vi "Point Dispense.vi"() -> ()   [LabVIEW 2016]
uses:
  GitHub/UCSB-Gantry/V5/Drivers/Aerotech A3200/Motion/WaitSingle.vi
  GitHub/UCSB-Gantry/V5/Drivers/Aerotech A3200/Aerotech VIs.lvlib
  GitHub/UCSB-Gantry/V5/Drivers/EFD Ultimus V/EFD Ultimus V.lvlib
panel:
  in  "stop":bool
  in  "Size of Square":dbl
  in  "Centerpoint":dbl[](array[numeric])
  in  "Go":bool
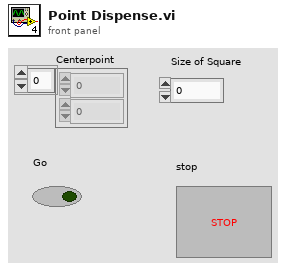
[diagram p1: front panel]
types:
  T1 = cluster{"Baud Rate ":u32, "Parity ":u16, "Data Bits ":u16, "Stop Bits":u16}
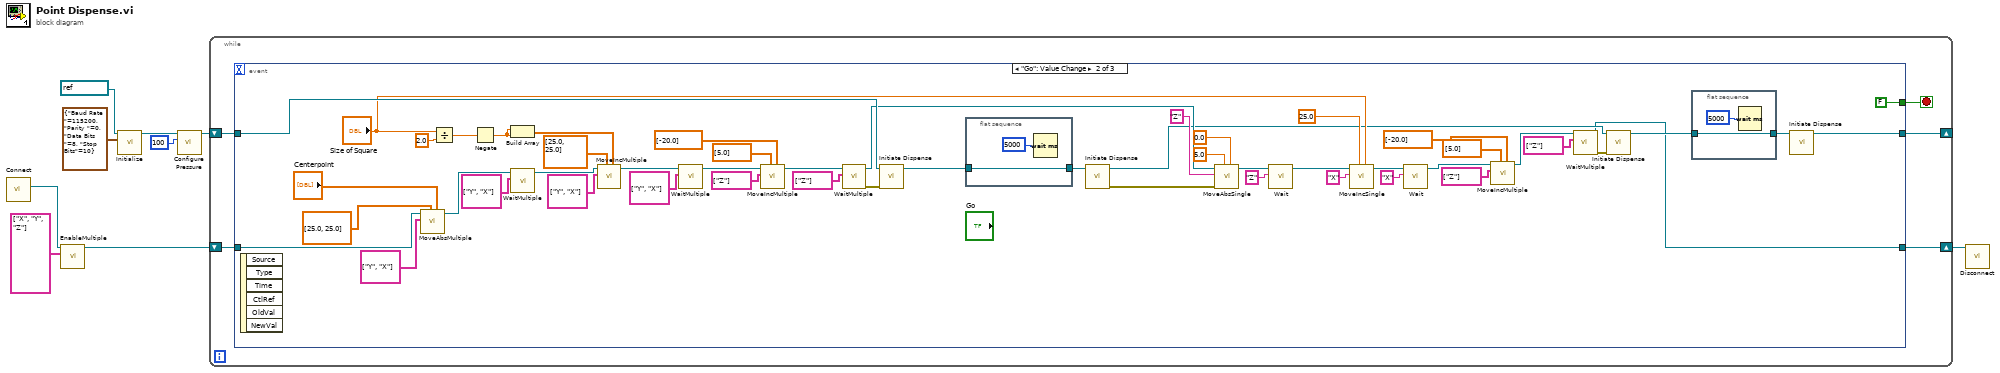
[diagram p0: block diagram]
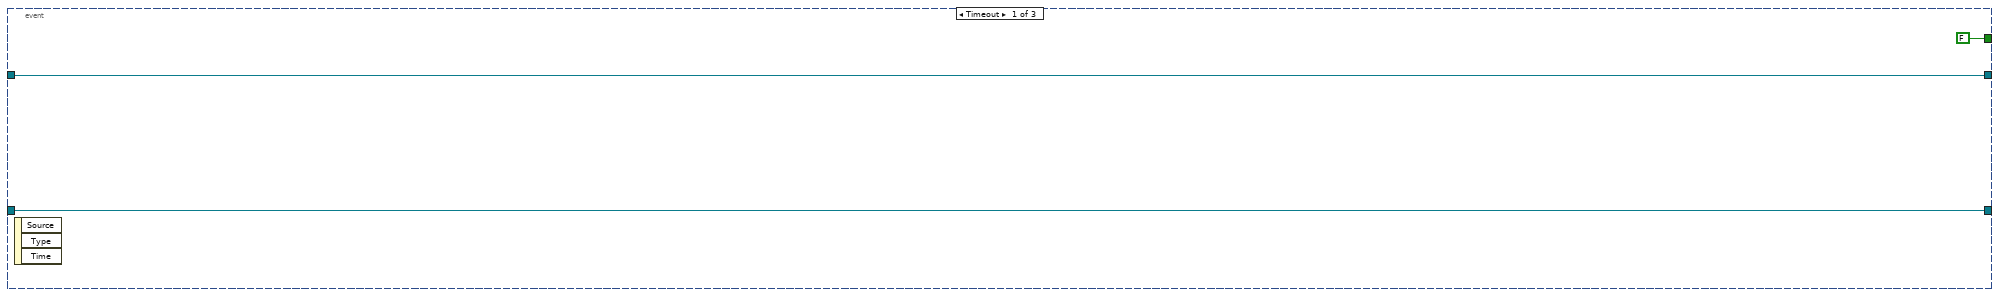
[diagram p2: hidden frame]
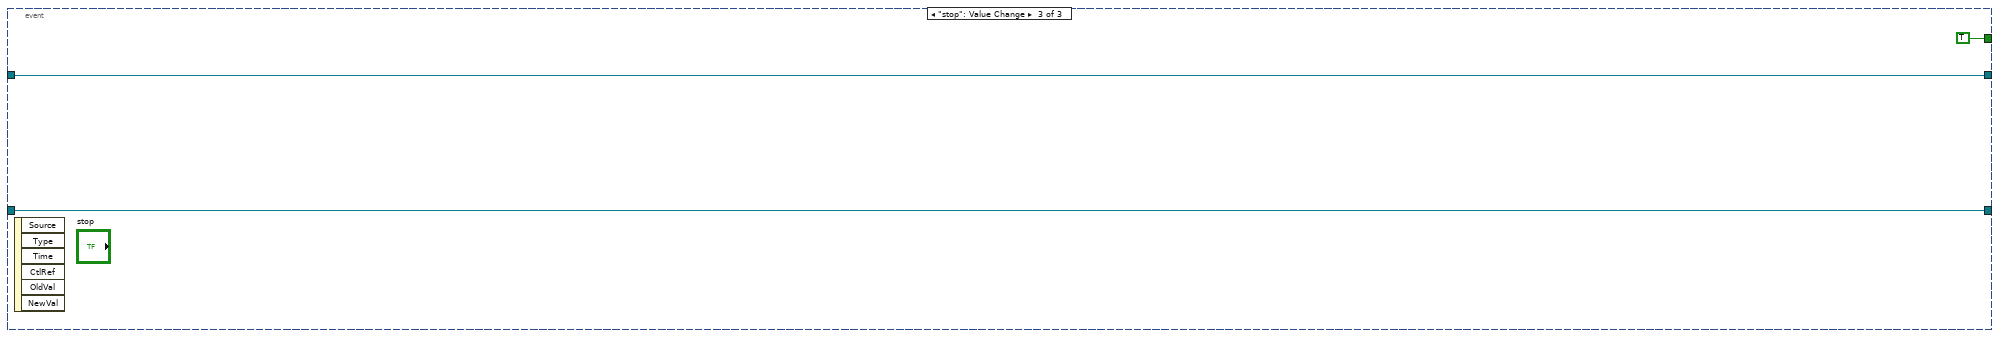
[diagram p3: hidden frame]
diagram:
  n1 = call "Connect.vi"() -> ("controller"=w9:refnum<k24>)  [unwired: 10 in, 1 out]
  n2 = call "EnableMultiple.vi"("axis names"=string[] ["X", "Y", "Z"], "controller in"=w9) -> ("controller out"=w7:refnum<k24>)  [unwired: 8 in, 1 out]
  n3 = call "Initialize.vi"("Serial Configuration"=T1 {"Baud Rate "=115200, "Parity "=0, "Data Bits "=8, "Stop Bits"=10}, "VISA resource name"=refnum<visa-resource-name> "COM1") -> ("VISA resource name out"=w3:refnum<visa-resource-name>)  [unwired: 8 in, 1 out]
  n4 = call "Configure Pressure.vi"("Pressure Setting (0000)"=i64 100, "VISA resource name"=w3) -> ("VISA resource name out"=w1:refnum<visa-resource-name>)  [unwired: 8 in, 1 out]
  n5 = while {
    shift-right: [w13] -> w6
    shift-left: w7 -> [w14]
    shift-right: [w10] -> _
    shift-left: w1 -> [w11]
    stop <- w12 stop-if-true
    n6 = event shown="[1] \"Go\": Value Change" {
      selector: _ -> [_ _ _]
      dyn-events: _ -> [_ _ _]
      timeout: _ -> [_ _ _]
      tunnel: w14 -> [w17 w66 w74]
      tunnel: [w17 w18 w74] -> w13
      tunnel: [FALSE FALSE TRUE] -> w12
      tunnel: w11 -> [w15 w46 w73]
      tunnel: [w15 w19 w73] -> w10
      event Timeout {
        n7 = event-data() -> ()  [unwired: 1 in, 3 out]
      }
      event "Go": Value Change {
        n8 = event-data() -> ()  [unwired: 1 in, 6 out]
        n9 = call "MoveAbsMultiple.vi"("positions"="Centerpoint", "speeds"=dbl[] [25.0, 25.0], "axis names"=string[] ["Y", "X"], "controller in"=w66) -> ("controller out"=w64:refnum<k24>)  [unwired: 6 in, 1 out]
        n10 = Divide(x="Size of Square", y=2.0) -> (x/y=w60:dbl)
        n11 = Negate(x=w60) -> (-x=w58:dbl)
        n12 = Build Array(w58, w58) -> (w57:dbl[])
        n13 = call "WaitMultiple.vi"("axis names"=string[] ["Y", "X"], "controller in"=w64) -> ("controller out"=w62:refnum<k24>)  [unwired: 7 in, 2 out]
        n14 = call "MoveIncMultiple.vi"("distances"=w57, "speeds"=dbl[] [25.0, 25.0], "axis names"=string[] ["Y", "X"], "controller in"=w62) -> ("controller out"=w54:refnum<k24>)  [unwired: 6 in, 1 out]
        n15 = call "WaitMultiple.vi"("axis names"=string[] ["Y", "X"], "controller in"=w54) -> ("controller out"=w52:refnum<k24>)  [unwired: 7 in, 2 out]
        n16 = call "MoveIncMultiple.vi"("distances"=dbl[] [-20.0], "speeds"=dbl[] [5.0], "axis names"=string[] ["Z"], "controller in"=w52) -> ("controller out"=w48:refnum<k24>)  [unwired: 6 in, 1 out]
        n17 = call "WaitMultiple.vi"("axis names"=string[] ["Z"], "controller in"=w48) -> ("error out"=w43:errorcluster, "controller out"=w42:refnum<k24>)  [unwired: 7 in, 1 out]
        n18 = call "Initiate Dispense.vi"("error in (no error)"=w43, "VISA resource name"=w46) -> ("VISA resource name out"=w45:refnum<visa-resource-name>)  [unwired: 8 in, 1 out]
        n19 = flat-sequence {
          tunnel: w45 -> [w71]
          tunnel: [w71] -> w44
          frame #0 {
            n20 = Wait (ms)(milliseconds to wait=u32 5000) -> ()  [unwired: 1 out]
          }
        }
        n21 = call "Initiate Dispense.vi"("VISA resource name"=w44) -> ("error out"=w41:errorcluster, "VISA resource name out"=w20:refnum<visa-resource-name>)  [unwired: 9 in]
        n22 = call "MoveAbsSingle.vi"("position"=0.0, "speed"=5.0, "error in (no error)"=w41, "axis name"="Z", "controller in"=w42) -> ("controller out"=w37:refnum<k24>)  [unwired: 5 in, 1 out]
        n23 = call-poly "Wait.vi"("axis name"="Z", "controller in"=w37) -> ("controller out"=w35:refnum<k24>)  [unwired: 7 in, 2 out]
        n24 = call "MoveIncSingle.vi"("distance"="Size of Square", "speed"=25.0, "axis name"="X", "controller in"=w35) -> ("controller out"=w31:refnum<k24>)  [unwired: 6 in, 1 out]
        n25 = call-poly "Wait.vi"("axis name"="X", "controller in"=w31) -> ("controller out"=w21:refnum<k24>)  [unwired: 7 in, 2 out]
        n26 = call "MoveIncMultiple.vi"("distances"=dbl[] [-20.0], "speeds"=dbl[] [5.0], "axis names"=string[] ["Z"], "controller in"=w21) -> ("controller out"=w26:refnum<k24>)  [unwired: 6 in, 1 out]
        n27 = call "WaitMultiple.vi"("axis names"=string[] ["Z"], "controller in"=w26) -> ("error out"=w22:errorcluster, "controller out"=w18:refnum<k24>)  [unwired: 7 in, 1 out]
        n28 = call "Initiate Dispense.vi"("error in (no error)"=w22, "VISA resource name"=w20) -> ("VISA resource name out"=w24:refnum<visa-resource-name>)  [unwired: 8 in, 1 out]
        n29 = flat-sequence {
          tunnel: w24 -> [w69]
          tunnel: [w69] -> w23
          frame #0 {
            n30 = Wait (ms)(milliseconds to wait=u32 5000) -> ()  [unwired: 1 out]
          }
        }
        n31 = call "Initiate Dispense.vi"("VISA resource name"=w23) -> ("VISA resource name out"=w19:refnum<visa-resource-name>)  [unwired: 9 in, 1 out]
      }
      event "stop": Value Change {
        n32 = event-data() -> ()  [unwired: 1 in, 6 out]
      }
    }
  }
  n33 = call "Disconnect.vi"("controller"=w6) -> ()  [unwired: 10 in, 1 out]
